vi "Master_ForceIdle.vi"(8 "error in":errorcluster, 10 "Actuators in":T1, 11 "State In":T2) -> (0 "error out":errorcluster, 2 "Actuators out":T1, 3 "State Out":T2)   [LabVIEW 2018]
doc: "Change the next state to Idle and deactivate all actuators to return the system to idle."
uses:
  TypeDef_ControlState.ctl
  Control/TypeDef_DigitalOuts.ctl
  Control/RunTypesLibrary/RunTypeList.ctl
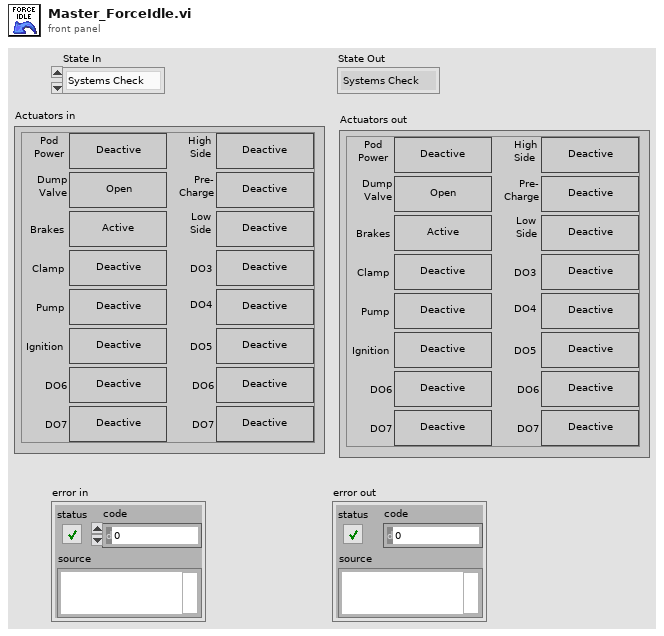
[diagram p1: front panel]
types:
  T1 = typedef "TypeDef_DigitalOuts.ctl" = cluster{"Pod Power":bool, "Dump Valve":bool, "Brakes":bool, "Clamp":bool, "Pump":bool, "Ignition":bool, "DO6":bool, "DO7":bool, "HighSide":bool, "Precharge":bool, "LowSide":bool, "DO3":bool, "DO4":bool, "DO5":bool, "DO62":bool, "DO72":bool}
  T2 = typedef "TypeDef_ControlState.ctl" = enum16{"Systems Check", "Idle", "Ready", "Pushing", "Coast", "Braking", "Fault", "Shutdown", "Service", "Precharge", "Blank"}
  T3 = typedef "RunTypeList.ctl" = enum16{"Full Run", "Systems Check", "Service"}
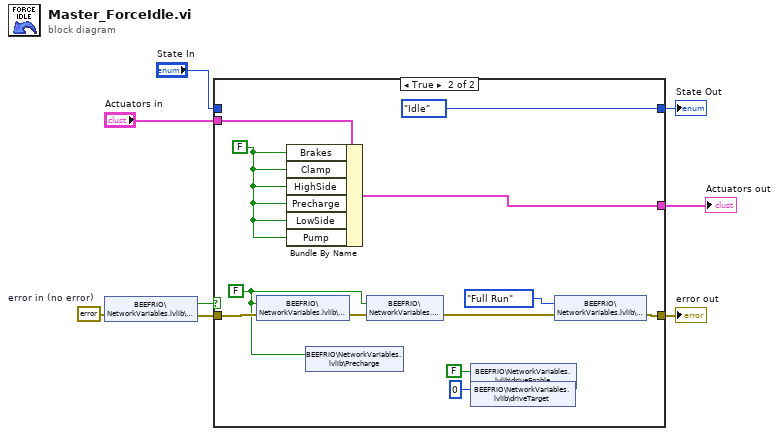
[diagram p0: block diagram]
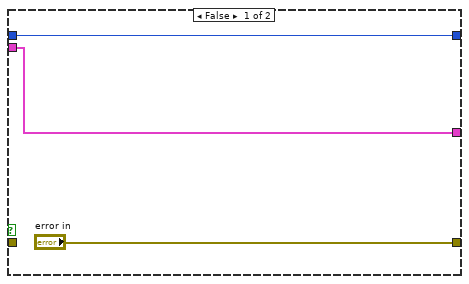
[diagram p2: hidden frame]
diagram:
  w2 = errorcluster {"status"=FALSE, "code"=0, "source"=""}  # error in (no error)
  n1 = shared-variable "BEEFRIO\\NetworkVariables.lvlib\\ForceIdle"(error in=w2) -> (w8:bool, error out=w1:errorcluster)
  n2 = case shown="True" w8 {
    tunnel: w1 -> [_ w20]
    tunnel: ["error in" w17] -> w7
    tunnel: [w11 TypeDef_ControlState."Idle" ("element")] -> w5
    tunnel: "State In" -> [w11 _]
    tunnel: "Actuators in" -> [w10 w21]
    tunnel: [w10 w22] -> w4
    frame False {
    }
    frame True {
      w14 = FALSE ("Brakes")
      w15 = FALSE ("Force Idle")
      n3 = shared-variable "BEEFRIO\\NetworkVariables.lvlib\\ForceIdle"(w15, error in=w20) -> (error out=w19:errorcluster)
      n4 = Bundle By Name(cluster=w21, "Brakes"=w14, "Clamp"=w14, "HighSide"=w14, "Precharge"=w14, "LowSide"=w14, "Pump"=w14) -> (w22:T1)
      n5 = shared-variable "BEEFRIO\\NetworkVariables.lvlib\\Precharge"(w15) -> ()  [unwired: 1 in, 1 out]
      n6 = shared-variable "BEEFRIO\\NetworkVariables.lvlib\\Ready"(w15, error in=w19) -> (error out=w18:errorcluster)
      n7 = shared-variable "BEEFRIO\\NetworkVariables.lvlib\\driveEnable"(FALSE ("driveEnable")) -> ()  [unwired: 1 in, 1 out]
      n8 = shared-variable "BEEFRIO\\NetworkVariables.lvlib\\driveTarget"(i16 0 ("driveTarget")) -> ()  [unwired: 1 in, 1 out]
      n9 = shared-variable "BEEFRIO\\NetworkVariables.lvlib\\RunType"(RunTypeList."Full Run" ("RunType"), error in=w18) -> (error out=w17:errorcluster)
    }
  }
  "error out" <- w7
  "State Out" <- w5
  "Actuators out" <- w4
